vi "Create States.vi"(5 "Sequencer":refnum<class "MessageQ.lvclass">, 6 "State Control":T1, 7 "VolatusAPI":refnum<class "VolatusAPI.lvclass">, 8 "error in (no error)":refnum<class "MultiErrors.lvclass">, 10 "Sequence Config":refnum<class "Sequence Config.lvclass">) -> (0 "error out":refnum<class "MultiErrors.lvclass">, 2 "States":map{string, refnum<class "State.lvclass">}(c390))   [LabVIEW 2020, in "VolatusSeq.lvlib" / "Sequence.lvclass"]
uses:
  Sequence.lvclass
  Sequence.lvclass/Sequence.ctl
  VolatusSeqConfig/Sequence Config/Sequence Config.lvclass
  State/State.lvclass
  VolatusErrorUtilities/MultiErrors/MultiErrors.lvclass
  Volatus/VolatusAPI/VolatusAPI.lvclass
  Sequence Time.ctl
  VolatusSeq.lvlib
  State Control.ctl
  Volatus/MessageQ/MessageQ.lvclass
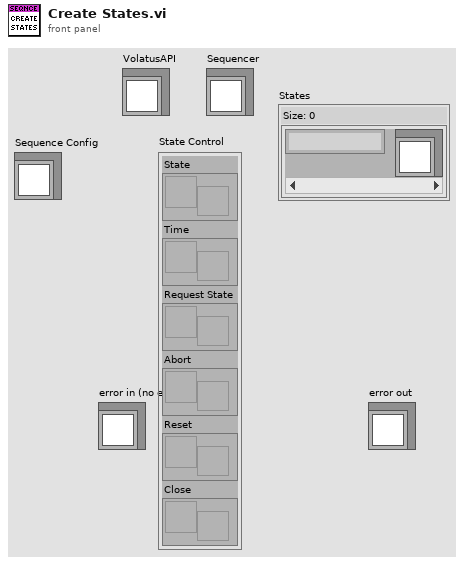
[diagram p1: front panel]
types:
  T1 = typedef "VolatusSeq.lvlib/State Control.ctl" = cluster{"State":refnum<notifier>, "Time":refnum<notifier>, "Request State":refnum<notifier>, "Abort":refnum<notifier>, "Reset":refnum<notifier>, "Close":refnum<notifier>}
  T2 = typedef "VolatusSeqConfig.lvlib/State.ctl" = cluster{"Name":string, "Steps":T3[], "Transitions":refnum<class "Transition Config.lvclass">[], "Comment":string, "Color":string, "Seq Name":string, "Report Conditions":bool}
  T3 = typedef "VolatusSeqConfig.lvlib/Step.ctl" = cluster{"Time":dbl, "Commands":refnum<class "Command Config.lvclass">[]}
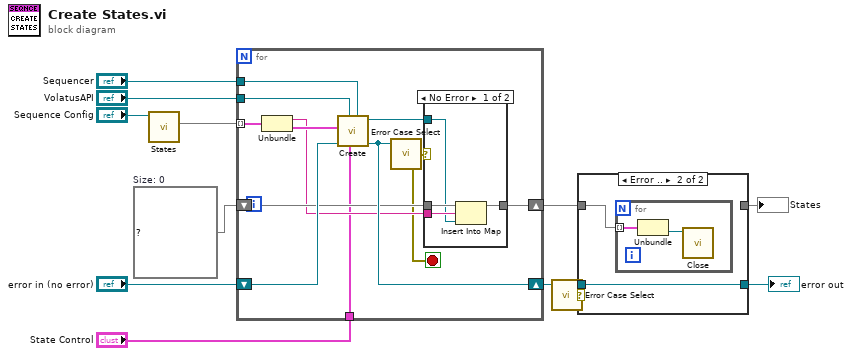
[diagram p0: block diagram]
diagram:
  w9 = map{string, refnum<class "State.lvclass">} {}  # Size: 0
  n1 = call "States.vi"("Sequence Config in"="Sequence Config") -> ("States"=w13:map{string, T2})  [unwired: 8 in, 2 out]
  n2 = for {
    tunnel: w13 -> [w23] mode=indexing
    tunnel: "VolatusAPI" -> [w21]
    shift-right: [w19] -> w11
    shift-left: w9 -> [w20]
    tunnel: "State Control" -> [w16]
    shift-right: [w25] -> w5
    shift-left: "error in (no error)" -> [w24]
    tunnel: "Sequencer" -> [w14]
    stop <- w15 stop-if-true
    n3 = Unbundle(w23) -> ("Name"=w18:string, "Info"=w22:T2)
    n4 = call "Create.vi"("Sequencer"=w14, "State Control"=w16, "VolatusAPI"=w21, "error in (no error)"=w24, "State"=w22) -> ("error out"=w25:refnum<class "MultiErrors.lvclass">, "State out"=w17:refnum<class "State.lvclass">)  [unwired: 5 in]
    n5 = call "Error Case Select.vi"("MultiErrors in"=w25) -> ("error out"=w15:errorcluster)  [unwired: 7 in, 1 out]
    n6 = case shown="No Error" w15 {
      tunnel: w20 -> [w29 w30]
      tunnel: [w28 w30] -> w19
      tunnel: w18 -> [w27 _]
      tunnel: w17 -> [w26 _]
      frame No Error {
        n7 = Insert Into Map(map in=w29, key=w27, value=w26) -> (map out=w28:map{string, refnum<class "State.lvclass">})  [unwired: 2 out]
      }
      frame Error {
      }
    }
  }
  n8 = call "Error Case Select.vi"("MultiErrors in"=w5) -> ("MultiErrors out"=w4:refnum<class "MultiErrors.lvclass">, "error out"=w3:errorcluster)  [unwired: 7 in]
  n9 = case shown="Error .." w3 {
    tunnel: w11 -> [w32 w34]
    tunnel: [w32 _] -> w10
    tunnel: w4 -> [w31 w33]
    tunnel: [w31 w33] -> w6
    frame No Error {
    }
    frame Error {
      n10 = for {
        tunnel: w34 -> [w36] mode=indexing
        n11 = Unbundle(w36) -> ("State out"=w35:refnum<class "State.lvclass">)  [unwired: 1 out]
        n12 = call "Close.vi"("State in"=w35) -> ()  [unwired: 10 in, 1 out]
      }
    }
  }
  "error out" <- w6
  "States" <- w10
